vi "Get Display String.vi"(11 "Int LT in":refnum<class "Int LT.lvclass">) -> (2 "Display String":string)   [LabVIEW 2018, in "Int LT.lvclass"]
uses:
  Int LT.lvclass
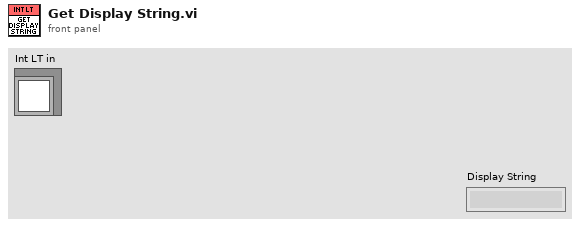
[diagram p1: front panel]
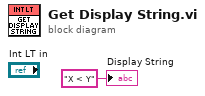
[diagram p0: block diagram]
diagram:
  "Display String" <- "X < Y" ("Display String")
